vi "Robot_0.vi"() -> ()   [LabVIEW 2015]
panel:
  in  "Tab Control":enum32{"Page 1"}(tab)
  out "Gauge":dbl(knob) scale=0.0..2.0
  out "Boolean":bool
  out "Boolean 2":bool
  out "Boolean 3":bool
  out "Boolean 4":bool
  out "Boolean 5":bool
  out "Boolean 6":bool
  out "Boolean 7":bool
  in  "stop":bool
  # "Robot"
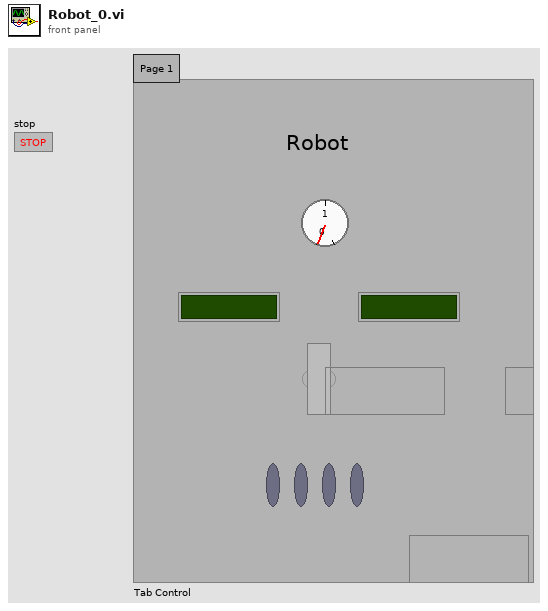
[diagram p1: front panel]
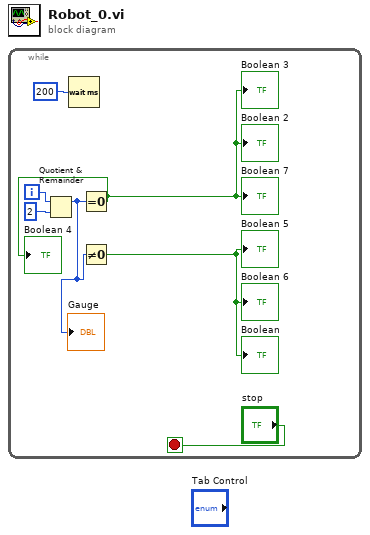
[diagram p0: block diagram]
diagram:
  n1 = while {
    i -> [w5]
    stop <- "stop" stop-if-true
    n2 = Quotient & Remainder(x=w5, y=2) -> (x-y*floor(x/y)=w1:i32)  [unwired: 1 out]
    "Gauge" <- w1
    n3 = Wait (ms)(milliseconds to wait=u32 200) -> ()  [unwired: 1 out]
    n4 = Equal To 0?(x=w1) -> (x = 0?=→"Boolean 2" →"Boolean 3" →"Boolean 4" →"Boolean 7":bool)
    n5 = Not Equal To 0?(x=w1) -> (x != 0?=→"Boolean" →"Boolean 5" →"Boolean 6":bool)
  }
